vi "CameraSetParams.vi"(8 "error in (no error)":errorcluster, 10 "settings":T2={"exposure"=0.0, "external"=FALSE, "roi"={"left"=0, "top"=0, "right"=0, "bottom"=0}, "frames"=0, "binning"={"x"=1, "y"=1}}, 11 "AndorSDK3 in":refnum<class "Andor3.lvclass">) -> (0 "error out":errorcluster, 1 "roi_out":T1, 2 "attributes":variant[](array[variant]), 3 "AndorSDK3 out":refnum<class "Andor3.lvclass">)   [LabVIEW 2010, in "Andor3.lvclass"]
uses:
  <userlib>/BIAS2/classes/Andor3/Andor3.lvclass
  <userlib>/BIAS2/subvis/ExposureSettings.ctl
  <userlib>/bias2/subvis/ROI_rect.ctl
  <userlib>/BIAS2/classes/Andor3/Andor3.lvclass/Andor3.ctl
  <userlib>/atcoreA/atcoreA.lvlib
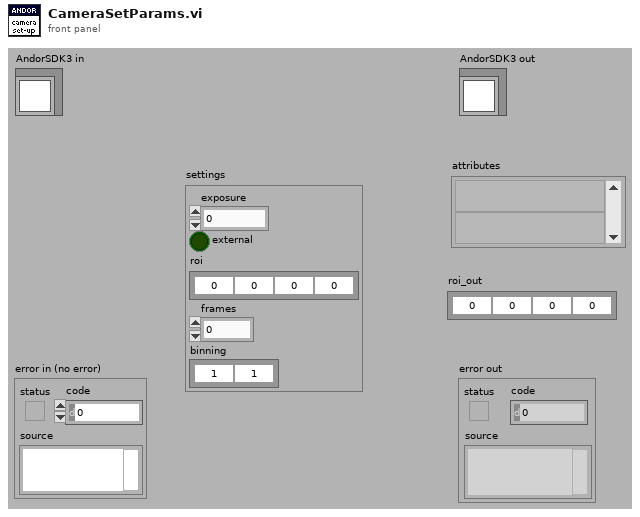
[diagram p1: front panel]
types:
  T1 = typedef "ROI_rect.ctl" = cluster{"left":i32, "top":i32, "right":i32, "bottom":i32}
  T2 = typedef "ExposureSettings.ctl" = cluster{"exposure":dbl, "external":bool, "roi":T1, "frames":i32, "binning":cluster{"x":u8, "y":u8}}
  T3 = cluster{"left":i32, "top":i32, "right":i32, "bottom":i32}
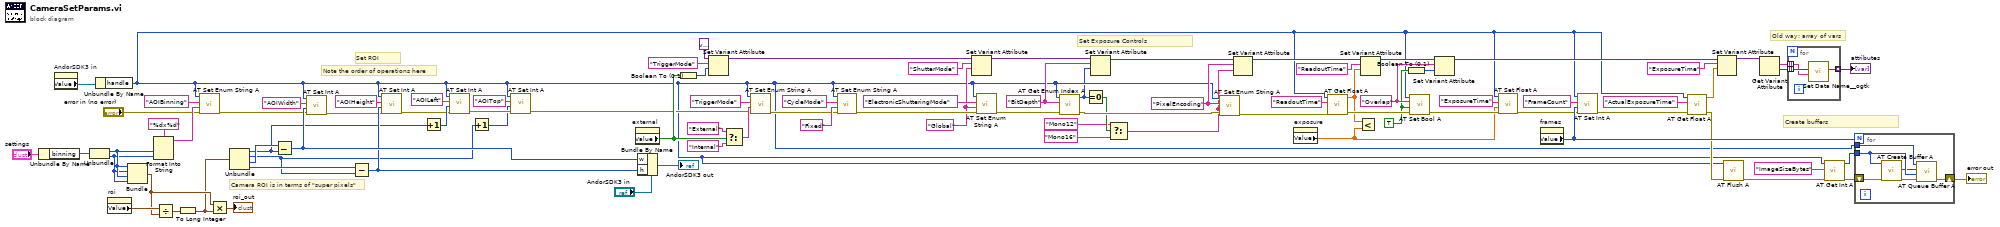
[diagram p0: block diagram]
diagram:
  w28 = TRUE ("Value")
  w29 = "PixelEncoding" ("Feature")
  w14 = "BitDepth" ("Feature")
  w40 = "Overlap" ("Data Name")
  w65 = "Global" ("String")
  # "Camera ROI is in terms of \"super pixels\""
  # "Note the order of operations here"
  # "Create buffers"
  # "Set Exposure Controls"
  # "Set ROI"
  # "Old way: array of vars"
  n1 = Unbundle By Name("settings") -> ("binning"=w7:cluster{"x":u8, "y":u8})
  n2 = property on="AndorSDK3 in" class="LVClassControl (strict)"() -> ("Value"=w55:refnum<class "Andor3.lvclass">)  [unwired: 2 in, 2 out]
  n3 = Unbundle(w7) -> ("x"=w6:u8, "y"=w5:u8)
  n4 = Unbundle By Name(w55) -> ("handle"=w13:i32)
  n5 = property on="roi" class="Clust (strict)"() -> ("Value"=w21:T3)  [unwired: 2 in, 2 out]
  n6 = Bundle("x"=w6, "y"=w5, "x"=w6, "y"=w5) -> (w3:cluster{"x":u8, "y":u8, "x":u8, "y":u8})  [unwired: 1 in]
  n7 = Format Into String(format string="%dx%d", w6, w5) -> (resulting string=w22:string)  [unwired: 2 in, 1 out]
  n8 = Divide(x=w21, y=w3) -> (x/y=w4:cluster{dbl, dbl, dbl, dbl})
  n9 = To Long Integer(number=w4) -> (32bit integer=w2:cluster{i32, i32, i32, i32})
  n10 = call <userlib>:"AT Set Enum String A.vi"("error in (no error)"="error in (no error)", "String"=w22, "Feature"="AOIBinning", "Hndl"=w13) -> ("error out"=w19:errorcluster)  [unwired: 7 in]
  n11 = Multiply(x=w3, y=w2) -> (x*y=→"roi_out":cluster{i32, i32, i32, i32})
  n12 = Unbundle(w2) -> (w51:i32, w50:i32, w92:i32, w91:i32)
  n13 = Subtract(x=w92, y=w51) -> (x-y=w54:i32)
  n14 = call <userlib>:"AT Set Int A.vi"("error in (no error)"=w19, "Value"=w54, "Feature"="AOIWidth", "Hndl"=w13) -> ("error out"=w18:errorcluster)  [unwired: 7 in]
  n15 = Subtract(x=w91, y=w50) -> (x-y=w52:i32)
  n16 = call <userlib>:"AT Set Int A.vi"("error in (no error)"=w18, "Value"=w52, "Feature"="AOIHeight", "Hndl"=w13) -> ("error out"=w26:errorcluster)  [unwired: 7 in]
  n17 = Increment(x=w51) -> (x+1=w49:i32)
  n18 = call <userlib>:"AT Set Int A.vi"("error in (no error)"=w26, "Value"=w49, "Feature"="AOILeft", "Hndl"=w13) -> ("error out"=w82:errorcluster)  [unwired: 7 in]
  n19 = Increment(x=w50) -> (x+1=w48:i32)
  n20 = call <userlib>:"AT Set Int A.vi"("error in (no error)"=w82, "Value"=w48, "Feature"="AOITop", "Hndl"=w13) -> ("error out"=w17:errorcluster)  [unwired: 7 in]
  n21 = property on="external" class="Bool (strict)"() -> ("Value"=w70:bool)  [unwired: 2 in, 2 out]
  n22 = Bundle By Name(cluster="AndorSDK3 in", "w"=w54, "h"=w52) -> (→"AndorSDK3 out":refnum<class "Andor3.lvclass">)
  n23 = Boolean To (0,1)(Boolean=w70) -> (0, 1=w71:i16)
  n24 = Set Variant Attribute(Variant=variant ("variant"), name="TriggerMode" ("Data Name"), value=w71) -> (Variant out=w42:variant)  [unwired: 1 in, 2 out]
  n25 = Select(t="External" ("Feature"), s=w70, f="Internal" ("Feature")) -> (s? t:f=w89:string)
  n26 = call <userlib>:"AT Set Enum String A.vi"("error in (no error)"=w17, "String"=w89, "Feature"="TriggerMode", "Hndl"=w13) -> ("error out"=w45:errorcluster)  [unwired: 7 in]
  n27 = call <userlib>:"AT Set Enum String A.vi"("error in (no error)"=w45, "String"="Fixed", "Feature"="CycleMode", "Hndl"=w13) -> ("error out"=w67:errorcluster)  [unwired: 7 in]
  n28 = Set Variant Attribute(Variant=w42, name="ShutterMode", value=w65) -> (Variant out=w33:variant)  [unwired: 1 in, 2 out]
  n29 = call <userlib>:"AT Set Enum String A.vi"("error in (no error)"=w67, "String"=w65, "Feature"="ElectronicShutteringMode", "Hndl"=w13) -> ("error out"=w16:errorcluster)  [unwired: 7 in]
  n30 = call <userlib>:"AT Get Enum Index A.vi"("error in (no error)"=w16, "Feature"=w14, "Hndl"=w13) -> ("error out"=w15:errorcluster, "Value"=w11:i32)  [unwired: 7 in]
  n31 = Equal To 0?(x=w11) -> (x = 0?=w12:bool)
  n32 = Set Variant Attribute(Variant=w33, name=w14, value=w11) -> (Variant out=w30:variant)  [unwired: 1 in, 2 out]
  n33 = Select(t="Mono12" ("String"), s=w12, f="Mono16" ("String")) -> (s? t:f=w8:string)
  n34 = call <userlib>:"AT Set Enum String A.vi"("error in (no error)"=w15, "String"=w8, "Feature"=w29, "Hndl"=w13) -> ("error out"=w32:errorcluster)  [unwired: 7 in]
  n35 = Set Variant Attribute(Variant=w30, name=w29, value=w8) -> (Variant out=w31:variant)  [unwired: 1 in, 2 out]
  n36 = property on="exposure" class="DigNum (strict)"() -> ("Value"=w27:dbl)  [unwired: 2 in, 2 out]
  n37 = call <userlib>:"AT Get Float A.vi"("error in (no error)"=w32, "Feature"="ReadoutTime", "Hndl"=w13) -> ("error out"=w46:errorcluster, "Value"=w43:dbl)  [unwired: 7 in]
  n38 = Less?(x=w43, y=w27) -> ()  [unwired: 1 out]
  n39 = Set Variant Attribute(Variant=w31, name="ReadoutTime" ("Data Name"), value=w43) -> (Variant out=w41:variant)  [unwired: 1 in, 2 out]
  n40 = Boolean To (0,1)(Boolean=w28) -> (0, 1=w39:i16)
  n41 = call <userlib>:"AT Set Bool A.vi"("error in (no error)"=w46, "Value"=w28, "Feature"=w40, "Hndl"=w13) -> ("error out"=w44:errorcluster)  [unwired: 7 in]
  n42 = Set Variant Attribute(Variant=w41, name=w40, value=w39) -> (Variant out=w38:variant)  [unwired: 1 in, 2 out]
  n43 = call <userlib>:"AT Set Float A.vi"("error in (no error)"=w44, "Value"=w27, "Feature"="ExposureTime", "Hndl"=w13) -> ("error out"=w37:errorcluster)  [unwired: 7 in]
  n44 = property on="frames" class="DigNum (strict)"() -> ("Value"=w59:i32)  [unwired: 2 in, 2 out]
  n45 = call <userlib>:"AT Set Int A.vi"("error in (no error)"=w37, "Value"=w59, "Feature"="FrameCount", "Hndl"=w13) -> ("error out"=w79:errorcluster)  [unwired: 7 in]
  n46 = call <userlib>:"AT Get Float A.vi"("error in (no error)"=w79, "Feature"="ActualExposureTime", "Hndl"=w13) -> ("error out"=w34:errorcluster, "Value"=w73:dbl)  [unwired: 7 in]
  n47 = Set Variant Attribute(Variant=w38, name="ExposureTime" ("Data Name"), value=w73) -> (Variant out=w36:variant)  [unwired: 1 in, 2 out]
  n48 = call <userlib>:"AT Flush A.vi"("error in (no error)"=w34, "Hndl"=w13) -> ("error out"=w47:errorcluster)  [unwired: 9 in]
  n49 = Get Variant Attribute(Variant=w36) -> (names=w63:string[], values=w62:variant[])  [unwired: 3 in, 2 out]
  n50 = for {
    tunnel: w63 -> [w94] mode=indexing
    tunnel: w62 -> [w95] mode=indexing
    tunnel: [w93] -> w61 mode=indexing
    n51 = call <userlib>:"Set Data Name__ogtk.vi"("Data Name"=w94, "Data"=w95) -> ("Renamed Data"=w93:variant)  [unwired: 8 in, 1 out]
  }
  "attributes" <- w61
  n52 = call <userlib>:"AT Get Int A.vi"("error in (no error)"=w47, "Feature"="ImageSizeBytes", "Hndl"=w13) -> ("error out"=w58:errorcluster, "Value"=w57:i64)  [unwired: 7 in]
  n53 = for {
    N: w59 -> [_]
    tunnel: w13 -> [w100]
    shift-right: [w97] -> w56
    shift-left: w58 -> [w101]
    tunnel: w57 -> [w99]
    n54 = call <userlib>:"AT Create Buffer A.vi"("error in (no error)"=w101, "Size"=w99) -> ("error out"=w98:errorcluster, "Buffer"=w96:u64)  [unwired: 8 in]
    n55 = call <userlib>:"AT Queue Buffer A.vi"("error in (no error)"=w98, "PtrSize"=w99, "Ptr"=w96, "Hndl"=w100) -> ("error out"=w97:errorcluster)  [unwired: 7 in]
  }
  "error out" <- w56
